vi "Bertta_v09_0.vi"() -> ()   [LabVIEW 2015]
panel:
  out "Started:":string
  in  "SHUTDOWN":bool
  in  "MASTER CONTROL":bool
  in  "Tab Control":T1(tab)
  in  "Read Seq":bool
  in  "Save Seq":bool
  in  "Configuration file":path=path "C:/Users/shresplab/Desktop/BerttaConfiguration.lvm" caption="Filename"
  in  "OK Button 2":bool
  out "Boolean":bool
  in  "User (initials)":string
  in  "Project name":string
  in  "Description":string
  out "Output file":string
  out "Sensor OK 6":bool
  out "Sensor OK 5":bool
  out "Sensor OK 4":bool
  out "Sensor OK 3":bool
  in  "OK Button":bool
  in  "Add comment":string
  out "PUMP 1":bool
  out "Target amount":dbl
  out "Scale weight":dbl
  out "Amount now":dbl
  out "Flow rate":dbl
  out "Time to target":dbl format="%<%H:%M:%S>t"
  out "Current step":dbl
  out "Target amount":dbl
  out "Amount now":dbl
  out "Tr":dbl
  out "Tj in":dbl
  out "Tj out":dbl
  out "T set":dbl
  out "Current step":i32
  out "RPM":dbl
  out "Torque 2":dbl
  out "Waveform Chart 5":dynamicdata(graph)
  out "Waveform Chart 6":dynamicdata(graph)
  out "Waveform Chart 7":dynamicdata(graph)
  out "Amount now":dbl
  out "Target amount":dbl
  out "Current step":dbl
  out "Time to target":dbl format="%<%H:%M:%S>t"
  out "Flow rate":dbl
  out "Amount now":dbl
  out "Scale weight":dbl
  out "Target amount":dbl
  out "PUMP 2":bool
  in  "Tab Control 2":T2(tab)
  out "Waveform Chart 3":dynamicdata(graph)
  out "Waveform Chart 8":dynamicdata(graph)
  out "Waveform Chart 11":dynamicdata(graph)
  out "Waveform Chart 9":dynamicdata(graph)
  out "Table":string[][](table)=[["14.8.2017 18.06.59", "0,000000", "417,670000", "-0,150000", "1,000000", "22,220000", "23,366837", "23,574959", "23,985852", "23,690000", "240,000000", "4,000000", "0,000000", "397,000000", "-397,000000", "1,000000"], ["14.8.2017 18.07.06", "0,000000", "417,640000", "-0,120000", "1,000000", "22,220000", "23,763115", "23,906257", "23,985694", "23,680000", "240,000000", "4,000000", "0,000000", "397,000000", "-397,000000", "1,000000"], ["14.8.2017 18.07.13", "0,000000", "417,640000", "-0,120000", "1,000000", "22,220000", "23,965922", "24,013440", "23,984906", "23,670000", "240,000000", "4,100000", "3,000000", "397,000000", "-397,000000", "1,000000"], ["14.8.2017 18.07.21", "0,000000", "417,640000", "-0,120000", "1,000000", "22,220000", "23,943860", "23,900110", "23,987113", "23,670000", "240,000000", "4,000000", "0,000000", "397,000000", "-397,000000", "1,000000"], ["14.8.2017 18.07.28", "0,000000", "417,640000", "-0,120000", "1,000000", "22,220000", "23,736328", "23,600018", "23,989004", "23,660000", "240,000000", "4,000000", "0,000000", "397,000000", "-397,000000", "1,000000"], ["14.8.2017 18.07.36", "0,000000", "417,640000", "-0,120000", "1,000000", "22,220000", "23,480910", "23,324538", "23,991053", "23,660000", "240,000000", "4,000000", "0,000000", "397,000000", "-397,000000", "1,000000"], ["14.8.2017 18.07.43", "0,000000", "417,640000", "-0,120000", "2,000000", "22,220000", "23,195579", "23,008270", "23,999093", "23,650000", "240,000000", "4,000000", "0,000000", "397,000000", "-397,000000", "1,000000"], ["14.8.2017 18.07.51", "0,000000", "417,650000", "-417,650000", "1,000000", "22,220000", "22,862541", "22,649021", "24,003979", "23,650000", "240,000000", "4,000000", "0,000000", "397,000000", "-397,000000", "2,000000"], ["14.8.2017 18.07.58", "0,000000", "417,640000", "0,010000", "1,000000", "22,220000", "22,541353", "22,354878", "24,005398", "23,650000", "240,000000", "4,000000", "0,000000", "397,000000", "-397,000000", "1,000000"], ["14.8.2017 18.08.06", "0,000000", "417,640000", "0,010000", "1,000000", "22,220000", "22,347931", "22,253738", "24,007605", "23,640000", "240,000000", "4,100000", "0,000000", "397,000000", "-397,000000", "1,000000"], ["14.8.2017 18.08.13", "0,000000", "417,640000", "0,010000", "1,000000", "22,220000", "22,329030", "22,302102", "24,006028", "23,640000", "240,000000", "4,000000", "0,000000", "395,820000", "-395,820000", "1,000000"], ["14.8.2017 18.08.20", "0,000000", "417,640000", "0,010000", "1,000000", "22,220000", "22,466849", "22,511320", "24,002403", "23,630000", "240,000000", "4,000000", "0,000000", "395,830000", "-0,010000", "1,000000"], ["14.8.2017 18.08.28", "0,000000", "417,640000", "0,010000", "1,000000", "22,220000", "22,707062", "22,835101", "24,000984", "23,620000", "240,000000", "4,000000", "0,000000", "395,830000", "-0,010000", "1,000000"], ["14.8.2017 18.08.35", "0,000000", "417,640000", "0,010000", "1,000000", "22,220000", "23,054104", "23,232979", "24,001299", "23,600000", "240,000000", "4,000000", "0,000000", "395,830000", "-0,010000", "1,000000"], ["14.8.2017 18.08.43", "0,000000", "417,640000", "0,010000", "1,000000", "22,220000", "23,412371", "23,522793", "24,002560", "23,590000", "240,000000", "4,000000", "0,000000", "395,820000", "0,000000", "1,000000"], ["14.8.2017 18.08.51", "0,000000", "417,640000", "0,010000", "1,000000", "22,220000", "23,596247", "23,656125", "24,003821", "23,580000", "240,000000", "4,000000", "0,000000", "395,820000", "0,000000", "1,000000"]]
  in  "T ext / T ext 2":enum32{"External 1", "External 2"}(radio)
  out "Sensor OK":bool
  in  "T fail":dbl=20.0
  out "Boolean 12":bool
  out "Boolean 7":bool
  out "Boolean 6":bool
  out "Boolean 5":bool
  out "Boolean 4":bool
  in  "?":bool
  in  "T manual setpoint":dbl=20.0
  in  "Lauda port":dbl=9.0
  in  "Manual select":enum32{"Tr", "Tj"}(radio)
  in  "TempSeq":dbl[][](array[numeric])=[[20.0, 40.0, 1.0, 30.0], [40.0, 50.0, 1.0, 30.0], [50.0, 20.0, 1.0, 30.0], [20.0, 20.0, 0.0, 20.0], [20.0, 20.0, 0.0, 20.0], [20.0, 20.0, 1000.0, 20.0]]
  out "T control":dbl
  out "Tr":dbl
  out "Tj in":dbl
  out "Tj out":dbl
  out "DT":dbl
  out "Elapsed":i32 format="%<%H:%M:%S>T"
  in  "PAUSE":bool
  out "Boolean 19":bool
  in  "Reset":bool
  in  "Treshold (Tset)":dbl=1.0
  in  "Tmax":dbl=199.0
  in  "Tmin":dbl=20.0
  out "Waveform Chart":dynamicdata(graph)
  out "T external 2":dbl
  in  "Xe":dbl=1.0
  in  "Ring":u16(ring) items=["SCALE 1", "SCALE 2", "SCALE 3"]
  out "Data out":dbl
  out "Port":i32=10
  in  "Radio Buttons":enum32{"Reglo Digital", "Reglo Analog", "PAM"}(radio)=enum."Reglo Analog"
  out "Speed":dbl
  out "mA":dbl format="%#_2g"
  in  "Port":i32=16
  out "RPM":dbl format="%#_2g"
  out "Boolean 18":bool
  out "Boolean 17":bool
  out "Boolean 16":bool
  out "Boolean 15":bool
  out "Boolean 14":bool
  out "Boolean 13":bool
  out "Boolean 11":bool
  out "Boolean 10":bool
  out "Boolean 9":bool
  out "Boolean 8":bool
  in  "PumpSeq":dbl[][](array[numeric])=[[3.0, 3.0, 7.0], [2.0, 2.0, 2.0], [4.0, 2.0, 100.0], [0.0, 0.0, 0.0], [0.0, 0.0, 0.0], [0.0, 0.0, 0.0], [0.0, 0.0, 0.0], [0.0, 0.0, 0.0], [0.0, 0.0, 0.0], [0.0, 0.0, 0.0], [0.0, 1.0, 0.0]]
  in  "?":bool
  out "Flow rate (g/min)":dbl
  out "Time (min)":dbl
  out "Target (g)":dbl
  out "Scale reading":dbl
  out "Step amount now":dbl
  out "Time to target":dbl format="%<%H:%M:%S>t"
  in  "Grams / min":dbl
  out "Waveform Chart 2":dynamicdata(graph)
  in  "?":bool
  out "Total amount now":dbl
  out "Total time":dbl
  out "Total amount target":dbl
  out "Boolean 20":bool
  in  "Reset 2":bool
  out "Waveform Chart 10":dynamicdata(graph)
  in  "Reset 3":bool
  out "Boolean 31":bool
  out "Total amount target 2":dbl
  out "Total time 2":dbl
  out "Boolean 30":bool
  out "Boolean 29":bool
  out "Boolean 28":bool
  out "Boolean 27":bool
  out "Boolean 26":bool
  out "Boolean 25":bool
  out "Boolean 24":bool
  out "Boolean 23":bool
  out "Boolean 22":bool
  out "Boolean 21":bool
  in  "PumpSeq 2":dbl[][](array[numeric])=[[3.0, 3.0, 7.0], [2.0, 2.0, 2.0], [4.0, 2.0, 100.0], [0.0, 0.0, 0.0], [0.0, 0.0, 0.0], [0.0, 0.0, 0.0], [0.0, 0.0, 0.0], [0.0, 0.0, 0.0], [0.0, 0.0, 0.0], [0.0, 0.0, 0.0], [0.0, 1.0, 0.0]]
  in  "Ring 2":u16(ring)=1 items=["SCALE 1", "SCALE 2", "SCALE 3"]
  out "Data out 2":dbl
  out "Port 3":i32=10
  in  "Radio Buttons 2":enum32{"Reglo Digital", "Reglo Analog", "PAM"}(radio)
  out "RPM":dbl format="%#_2g"
  in  "Port":i32=15
  out "mA":dbl format="%#_2g"
  out "Speed":dbl
  in  "?":bool
  in  "Grams / min":dbl
  out "Time (min)":dbl
  out "Target (g)":dbl
  out "Total amount now":dbl
  out "Time to target":dbl format="%<%H:%M:%S>t"
  in  "?":bool
  out "Step amount now":dbl
  out "Scale reading":dbl
  out "Flow rate (g/min)":dbl
  in  "Bypass select 2":enum32{"Remote", "Manual"}(radio)
  in  "Port":dbl=13.0
  out "RPM":dbl
  out "Torque":dbl
  in  "Set RPM":dbl(slide) scale=0.0..500.0
  out "Waveform Chart 4":dynamicdata(graph)
  out "DAQ 9217 (PT100)":errorcluster
  # "PUMP & SCALE 1"
  # "PUMP & SCALE 2"
  # "STEP"
  # "STEP"
  # "TOTAL"
  # "TOTAL"
  # "Temperature sensor:"
  # "Manual control:"
  # "Tinit     >    Tset       Min. time      Tfail"
  # "Manual control / end of sequence"
  # "Manual control"
  # "Secondary temperature sensor"
  # "Device communication"
  # "Grams    /   min"
  # "End of sequence"
  # "Manual control"
  # "Device communication"
  # "Pump configuration"
  # "Scale configuration"
  # "Grams    /   min"
  # "End of sequence"
  # "Manual control"
  # "Device communication"
  # "Pump configuration"
  # "Scale configuration"
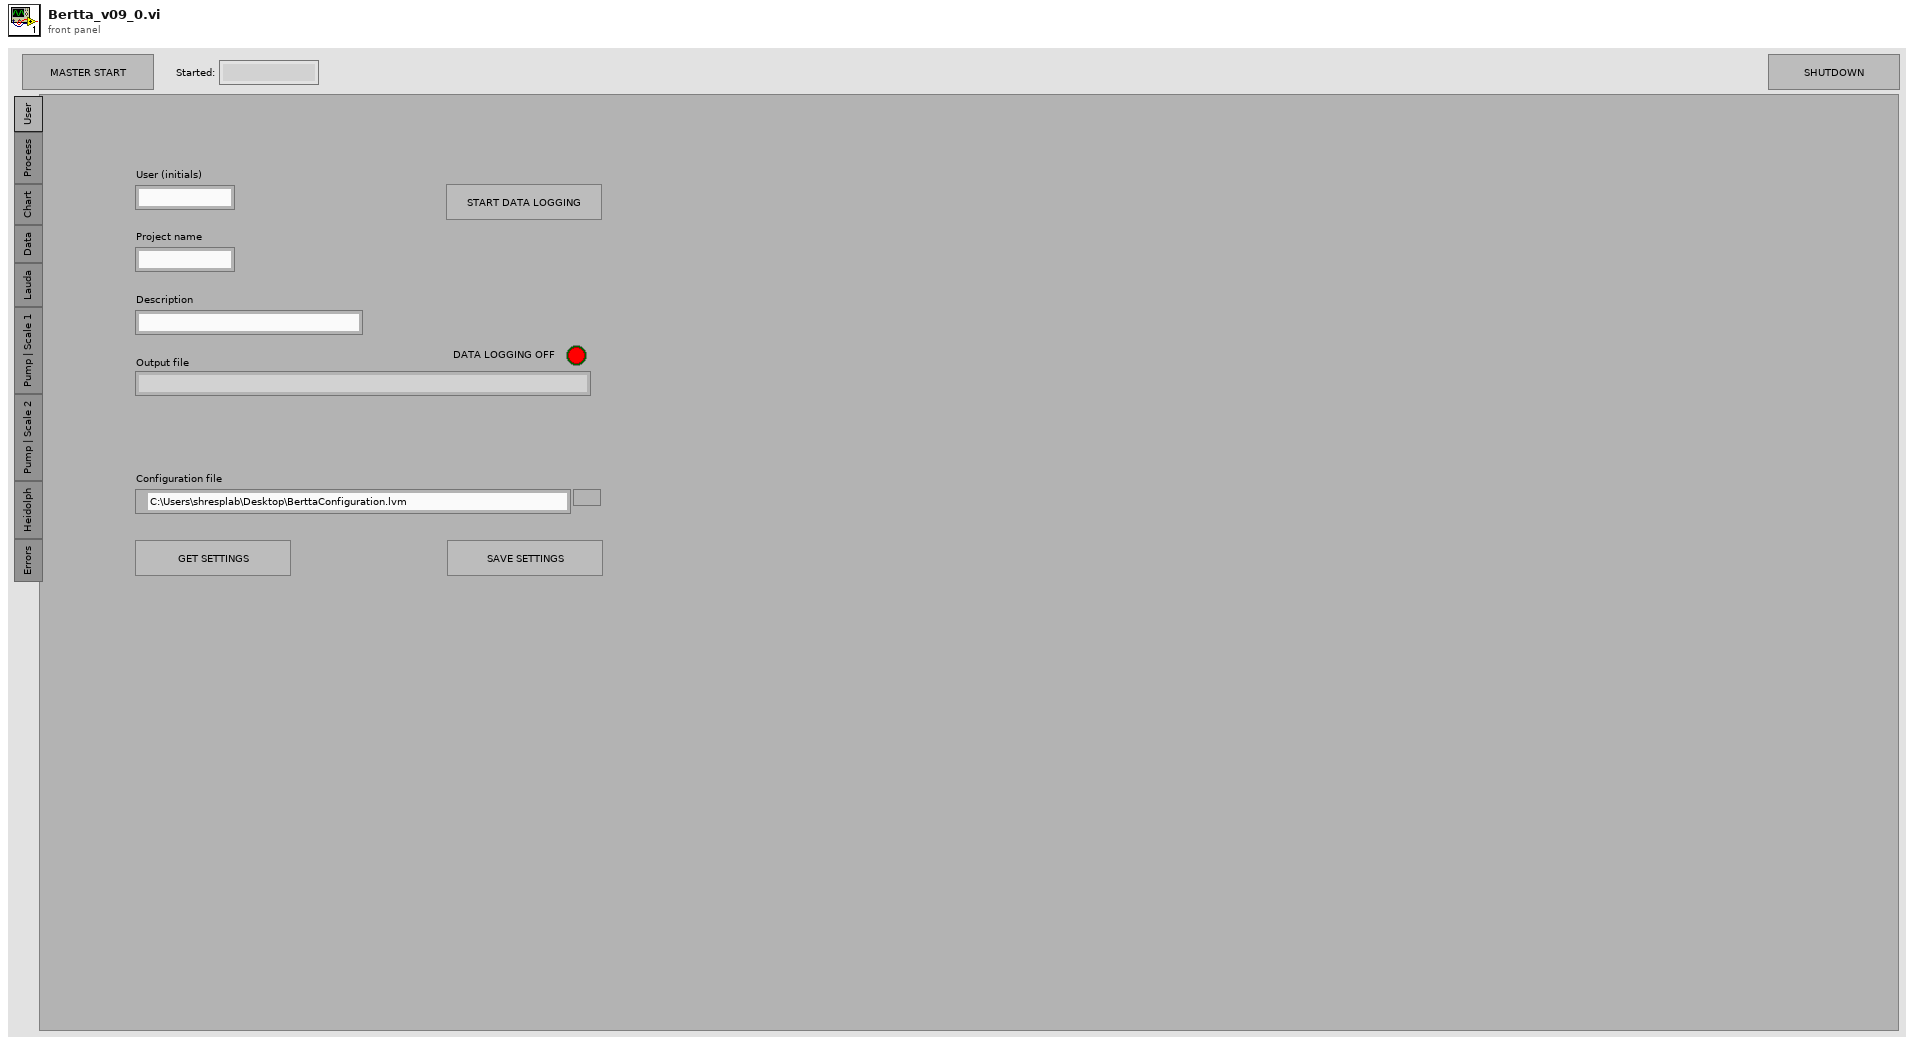
[diagram p1: front panel]
types:
  T1 = enum32{"User", "Process", "Chart", "Data", "Lauda", "Pump | Scale 1", "Pump | Scale 2", "Heidolph", "Errors"}
  T2 = enum32{"Temperatures", "Scale / Pump 1", "Scale / Pump 2", "RPM / torque"}
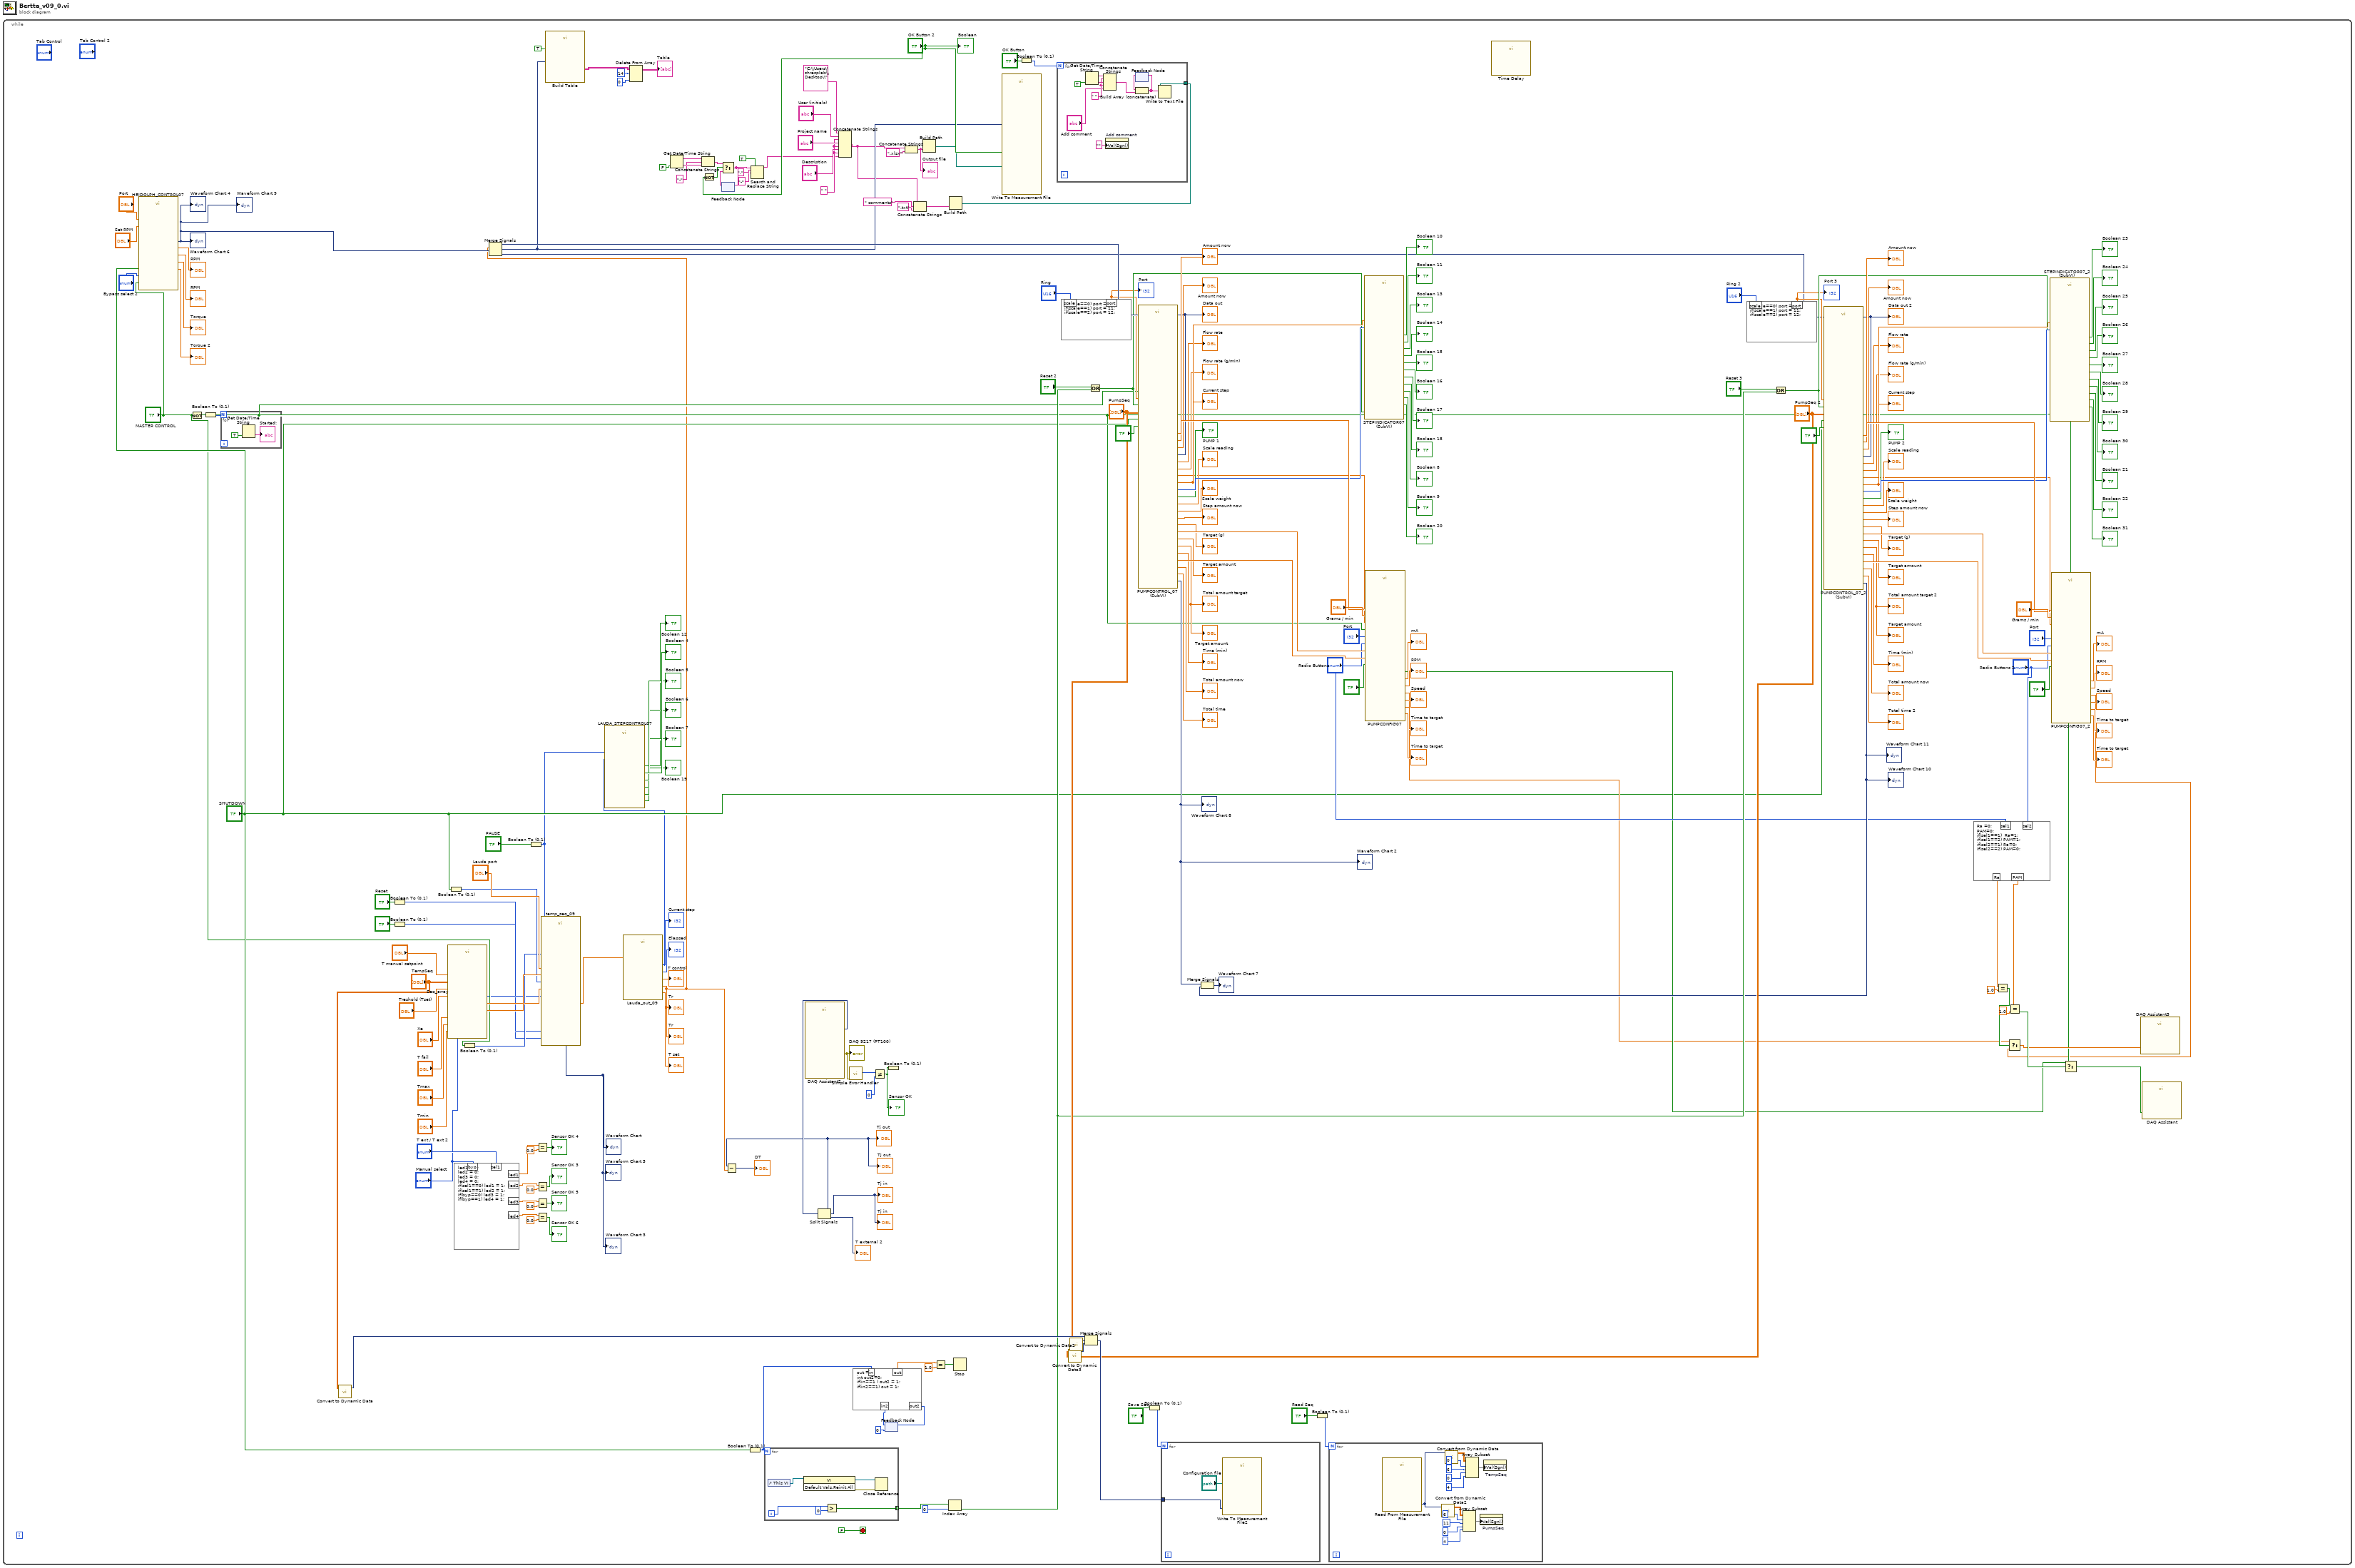
[diagram p0: block diagram]
diagram:
  n1 = while {
    stop <- FALSE stop-if-true
    w174 = " "
    n2 = call "HEIDOLPH_CONTROL07.vi"("master"="MASTER CONTROL", "shutdown"="SHUTDOWN", "Bypass select"="Bypass select 2", "Set RPM"="Set RPM", "Device port"="Port") -> ("Dynamic Data"=w185:dynamicdata, "RPM"=→"RPM":dbl, "RPM 2"=→"RPM":dbl, "Torque"=→"Torque":dbl, "Torque 2"=→"Torque 2":dbl)  [unwired: 2 in]
    "Waveform Chart 4" <- w185
    "Waveform Chart 6" <- w185
    "Waveform Chart 9" <- w185
    n3 = Not(x="MASTER CONTROL") -> (.not. x?=w165:bool)
    n4 = Boolean To (0,1)(Boolean=w165) -> (0, 1=w166:i16)
    n5 = for {
      N: w166 -> [_]
      n6 = Get Date/Time String(want seconds? (F)=TRUE) -> (time string=→"Started:":string)  [unwired: 2 in, 1 out]
    }
    n7 = call "Convert to Dynamic Data"("2D Array"="TempSeq") -> ("Dynamic Data Type"=w160:dynamicdata)  [unwired: 3 in]
    n8 = Boolean To (0,1)(Boolean="Reset") -> (0, 1=w13:i16)
    n9 = Boolean To (0,1)(Boolean="?") -> (0, 1=w15:i16)
    n10 = call "Seq_array.vi"("Tfail_manual"="T fail", "TempSeq in"="TempSeq", "Tmin"="Tmin", "Tmax"="Tmax", "Treshold (Tset)"="Treshold (Tset)", "T manual setpoint"="T manual setpoint", "Xe"="Xe") -> ("TimeParams"=w29:dbl[], "TempParams"=w30:dbl[])  [unwired: 3 in]
    n11 = Boolean To (0,1)(Boolean="SHUTDOWN") -> (0, 1=w25:i16)
    n12 = formula code="led1 = 0;\nled2 = 0;\nled3 = 0;\nled4 = 0;\nif(sel1==0) led1 = 1;\nif(sel1==1) led2 = 1;\nif(byp==0) led3 = 1;\nif(byp==1) led4 = 1;"("sel1"="T ext / T ext 2", "byp"="Manual select") -> ("led1"=w109:dbl, "led2"=w107:dbl, "led3"=w102:dbl, "led4"=w101:dbl)
    n13 = Boolean To (0,1)(Boolean="MASTER CONTROL") -> (0, 1=w23:i16)
    n14 = Boolean To (0,1)(Boolean="PAUSE") -> (0, 1=w19:i16)
    n15 = Equal?(x=w109, y=0.0) -> (x = y?=→"Sensor OK 4":bool)
    n16 = Equal?(x=w107, y=0.0) -> (x = y?=→"Sensor OK 3":bool)
    n17 = Equal?(x=w102, y=0.0) -> (x = y?=→"Sensor OK 5":bool)
    n18 = Equal?(x=w101, y=0.0) -> (x = y?=→"Sensor OK 6":bool)
    n19 = call "temp_seq_09.vi"("master"=w23, "shutdown"=w25, "Tr_orTj"="Manual select", "pause"=w19, "TempParams"=w30, "TimeParams"=w29, "port"="Lauda port", "reset"=w13, "manual"=w15) -> ("params"=w21:dbl[], "Waveform Chart"=→"Waveform Chart 3" →"Waveform Chart" →"Waveform Chart 5":dynamicdata)  [unwired: 3 in, 2 out]
    n20 = call "Lauda_out_09.vi"("params"=w21) -> ("Elapsed"=→"Elapsed":i32, "Tr"=w3:dbl, "Current step"=w2:i32, "T control"=→"T control":dbl, "T set"=→"T set":dbl)  [unwired: 6 in]
    "Tr" <- w3
    "Tr" <- w3
    "Current step" <- w2
    n21 = call "LAUDA_STEPCONTROL07.vi"("step"=w2, "pause"=w19) -> ("Boolean 13"=→"Boolean 19":bool, "Boolean 6"=→"Boolean 6":bool, "Boolean 5"=→"Boolean 5":bool, "Boolean 4"=→"Boolean 4":bool, "Boolean 7"=→"Boolean 7":bool, "Boolean 12"=→"Boolean 12":bool)  [unwired: 4 in]
    n22 = Get Date/Time String(want seconds? (F)=FALSE) -> (date string=w145:string, time string=w140:string)  [unwired: 2 in]
    n23 = Concatenate Strings(w145, "-" ("string"), w140) -> (w144:string)
    n24 = Not(x="OK Button 2") -> (.not. x?=w141:bool)
    n25 = feedback #1() -> (w143:string)  [unwired: 1 in]
    n26 = Select(t=w144, s=w141, f=w143) -> (s? t:f=w136:string)
    n27 = feedback-in #1(w136) -> ()
    n28 = Boolean To (0,1)(Boolean="SHUTDOWN") -> (0, 1=w115:i16)
    n29 = Search and Replace String(replace all?=TRUE ("replace all? (F)"), input string=w136, search string=".", replace string="-" ("replace string (\"\")")) -> (result string=w135:string)  [unwired: 4 in, 3 out]
    n30 = for {
      N: w115 -> [_]
      tunnel: [w254] -> w162 mode=indexing
      i -> [w256]
      n31 = control-ref of="This VI"() -> (w259:refnum<vi>)
      n32 = invoke class="VI" method="Default Vals.Reinit All"(reference=w259) -> (reference out=w257:refnum<vi>, error out=w258:errorcluster)  [unwired: 2 in, 1 out]
      n33 = Greater?(x=w256, y=0) -> (0:w254:bool)
      n34 = Close Reference(reference=w257, error in (no error)=w258) -> ()  [unwired: 1 out]
    }
    n35 = call "DAQ Assistant2"() -> ("data"=w8:dynamicdata, "error out"=w180:errorcluster)  [unwired: 17 in, 1 out]
    "DAQ 9217 (PT100)" <- w180
    n36 = Split Signals(w8) -> (w5:dynamicdata, →"Tj in" →"Tj in":dynamicdata, →"T external 2":dynamicdata)  [unwired: 3 in]
    "Tj out" <- w5
    "Tj out" <- w5
    n37 = Subtract(x=w5, y=w3) -> (x-y=→"DT":dynamicdata)
    n38 = Concatenate Strings("C:\\Users\\shresplab\\Desktop\\", "User (initials)", w174, "Project name", w174, "Description", w174, w135) -> (w125:string)
    n39 = call <vilib>:"Simple Error Handler.vi"("error in (no error)"=w180) -> ("code out"=w179:i32)  [unwired: 4 in, 4 out]
    n40 = Not Equal?(x=w179, y=0) -> (x != y?=w152:bool)
    "Sensor OK" <- w152
    n41 = feedback #2(0) -> (w113:i32)
    n42 = formula code="out = 0;\nint out2=0;\nif(in==1 ) out2 = 1;\nif(in2==1) out = 1;"("in"=w115, "in2"=w113) -> ("out"=w117:dbl, "out2"=w114:i32)
    n43 = feedback-in #2(w114) -> ()
    n44 = Boolean To (0,1)(Boolean=w152) -> ()  [unwired: 1 out]
    n45 = Concatenate Strings(w125, ".xlsx") -> (w128:string)
    "Output file" <- w128
    n46 = Concatenate Strings(w125, " comments" ("string"), ".txt" ("string")) -> (w122:string)
    n47 = Build Path(name or relative path=w128) -> (appended path=w126:path)  [unwired: 1 in]
    n48 = Equal?(x=w117, y=1.0) -> (x = y?=w116:bool)
    n49 = Index Array(array=w162, index=0) -> (element=w54:bool)
    n50 = Build Path(name or relative path=w122) -> (appended path=w121:path)  [unwired: 1 in]
    n51 = Stop(stop? (T)=w116) -> ()
    n52 = Boolean To (0,1)(Boolean="OK Button") -> (0, 1=w120:i16)
    n53 = for {
      N: w120 -> [_]
      tunnel: w121 -> [w231]
      w235 = " " ("string")
      n54 = Get Date/Time String(want seconds? (F)=TRUE) -> (date string=w238:string, time string=w236:string)  [unwired: 2 in]
      n55 = Concatenate Strings(w238, w235, w236, w235, "Add comment") -> (w234:string)
      n56 = property on="Add comment" class="Str"("Val(Sgnl)"="" ("Value (Signaling)")) -> ()  [unwired: 2 in, 2 out]
      n57 = feedback #3() -> (w233:string[])  [unwired: 1 in]
      n58 = Build Array (concatenate)(w233, w234) -> (w232:string[])
      n59 = feedback-in #3(w232) -> ()
      n60 = Write to Text File(file (use dialog)=w231, text=w232) -> ()  [unwired: 2 in, 3 out]
    }
    n61 = formula code="if(scale==0) port = 10;\nif(scale==1) port = 11;\nif(scale==2) port = 12;"("scale"="Ring") -> ("port"=w147:dbl)
    "Port" <- w147
    n62 = call "Convert to Dynamic Data3"("2D Array"="PumpSeq 2") -> ("Dynamic Data Type"=w53:dynamicdata)  [unwired: 3 in]
    n63 = call "Convert to Dynamic Data2"("2D Array"="PumpSeq") -> ("Dynamic Data Type"=w159:dynamicdata)  [unwired: 3 in]
    n64 = Merge Signals(w160, w159, w53) -> (w158:dynamicdata)
    n65 = Or(x="Reset 2", y=w54) -> (x .or. y?=w151:bool)
    n66 = call "PUMPCONTROL_07 (SubVI).vi"("Port"=w147, "Pause"="MASTER CONTROL", "Master start"="?", "shutdown"="SHUTDOWN", "Seq in"="PumpSeq", "reset"=w151) -> ("Amount now"=→"Amount now":dbl, "Amount now 2"=→"Amount now":dbl, "Flow rate out"=w170:dbl, "Step amount now"=→"Step amount now":dbl, "Total amount now"=→"Total amount now":dbl, "Total time"=→"Total time":dbl, "Numeric 2"=w223:i16, "PUMP 1"=→"PUMP 1":bool, "Numeric"=w220:dbl, "Flow rate"=→"Flow rate":dbl, "Dynamic Data"=w186:dynamicdata, "Target amount"=→"Target amount":dbl, "Time (min) 2"=w224:dbl, "Target amount 2"=→"Total amount target" →"Target amount":dbl, "Scale reading"=→"Scale reading":dbl, "Flow rate (g/min)"=→"Flow rate (g/min)":dbl, "Target (g) 2"=w225:dbl, "Target (g)"=→"Target (g)":dbl, "Time (min)"=→"Time (min)":dbl, "Waveform Chart 2"=w36:dynamicdata, "Scale weight"=→"Scale weight":dbl, "Amount (g)"=w226:dbl)
    "Waveform Chart 2" <- w36
    "Current step" <- w220
    "Data out" <- w186
    "Waveform Chart 8" <- w36
    n67 = Boolean To (0,1)(Boolean="Save Seq") -> (0, 1=w157:i16)
    n68 = for {
      N: w157 -> [_]
      tunnel: w158 -> [w253]
      n69 = call "Write To Measurement File2"("Signals"=w253, "Filename"="Configuration file") -> ()  [unwired: 15 in, 3 out]
    }
    n70 = Boolean To (0,1)(Boolean="Read Seq") -> (0, 1=w154:i16)
    n71 = for {
      N: w154 -> [_]
      n72 = call "Read From Measurement File"() -> ("Signals"=w241:dynamicdata)  [unwired: 6 in, 5 out]
      n73 = call "Convert from Dynamic Data2"("Dynamic Data Type"=w241) -> ("Array"=w240:dbl[][])  [unwired: 3 in]
      n74 = call "Convert from Dynamic Data"("Dynamic Data Type"=w241) -> ("Array"=w249:dbl[][])  [unwired: 3 in]
      n75 = Array Subset(array=w240, index (row)=6 ("index"), length (row)=11 ("length"), index (col)=0 ("index"), length (col)=4 ("length")) -> (w239:dbl[][])
      n76 = Array Subset(array=w249, index (row)=0 ("index"), length (row)=6 ("length"), index (col)=0 ("index"), length (col)=4 ("length")) -> (w246:dbl[][])
      n77 = property on="PumpSeq" class="Arr (strict)"("Val(Sgnl)"=w239) -> ()  [unwired: 2 in, 2 out]
      n78 = property on="TempSeq" class="Arr (strict)"("Val(Sgnl)"=w246) -> ()  [unwired: 2 in, 2 out]
    }
    n79 = call "STEPINDICATOR07 (SubVI).vi"("Numeric"=w220, "Numeric 2"=w223, "Reset"=w151) -> ("Boolean 18"=→"Boolean 18":bool, "Boolean 8"=→"Boolean 8":bool, "Boolean 9"=→"Boolean 9":bool, "Boolean 17"=→"Boolean 17":bool, "Boolean 10"=→"Boolean 10":bool, "Boolean 16"=→"Boolean 16":bool, "Boolean 11"=→"Boolean 11":bool, "Boolean 15"=→"Boolean 15":bool, "Boolean 14"=→"Boolean 14":bool, "Boolean 13"=→"Boolean 13":bool, "Boolean 19"=→"Boolean 20":bool)  [unwired: 2 in]
    n80 = call "PUMPCONFIG07.vi"(0:"?", "Radio Buttons"="Radio Buttons", "Bypass (g/min)"="Grams / min", "Target (g) in"=w225, "Amount (g)"=w226, "Time (min) in"=w224, "Flow rate in"=w170, "OK Button"="MASTER CONTROL", "Port"="Port") -> ("Time to target 2"=→"Time to target":dbl, "Time to target"=→"Time to target":dbl, "mA"=→"mA":dbl, "signal"=w40:dbl, "Speed"=→"Speed":dbl, "RPM"=→"RPM":dbl, "Array"=w42:bool[])
    n81 = call "Time Delay"() -> ()  [unwired: 11 in, 1 out]
    n82 = formula code="if(scale==0) port = 10;\nif(scale==1) port = 11;\nif(scale==2) port = 12;"("scale"="Ring 2") -> ("port"=w55:dbl)
    "Port 3" <- w55
    n83 = Or(x="Reset 3", y=w54) -> (x .or. y?=w58:bool)
    n84 = call "PUMPCONTROL_07_2 (SubVI).vi"("Port"=w55, "Pause"="MASTER CONTROL", "Master start"="?", "shutdown"="SHUTDOWN", "Seq in"="PumpSeq 2", "reset"=w58) -> ("Amount now"=→"Amount now":dbl, "Amount now 2"=→"Amount now":dbl, "Flow rate out"=w62:dbl, "Step amount now"=→"Step amount now":dbl, "Total amount now"=→"Total amount now":dbl, "Total time"=→"Total time 2":dbl, "Numeric 2"=w94:i16, "PUMP 1"=→"PUMP 2":bool, "Numeric"=w91:dbl, "Flow rate"=→"Flow rate":dbl, "Dynamic Data"=w34:dynamicdata, "Target amount"=→"Target amount":dbl, "Time (min) 2"=w95:dbl, "Target amount 2"=→"Total amount target 2" →"Target amount":dbl, "Scale reading"=→"Scale reading":dbl, "Flow rate (g/min)"=→"Flow rate (g/min)":dbl, "Target (g) 2"=w96:dbl, "Target (g)"=→"Target (g)":dbl, "Time (min)"=→"Time (min)":dbl, "Waveform Chart 2"=w51:dynamicdata, "Scale weight"=→"Scale weight":dbl, "Amount (g)"=w97:dbl)
    "Waveform Chart 10" <- w51
    "Current step" <- w91
    "Data out 2" <- w34
    "Waveform Chart 11" <- w51
    n85 = Merge Signals(w186, w3, w185, w34) -> (w132:dynamicdata)
    n86 = call "Build Table"("Include time data"=TRUE, "Signals"=w132) -> ("Table"=w131:string[][])  [unwired: 3 in, 6 out]
    n87 = Delete From Array(array=w131, length=14, index (col)=0 ("index (row)")) -> (array with subset deleted=→"Table":string[][])  [unwired: 1 in, 1 out]
    n88 = call "Write To Measurement File"("Signals"=w132, "Enable"="OK Button 2", "Filename"=w126) -> ()  [unwired: 14 in, 3 out]
    n89 = Merge Signals(w36, w51) -> (→"Waveform Chart 7":dynamicdata)
    n90 = formula code="Ra =0;\nPAM=0;\nif(sel1==1)  Ra=1;\nif(sel1==2) PAM=1;\nif(sel2==1) Ra=0;\nif(sel2==2) PAM=0;"("sel1"="Radio Buttons", "sel2"="Radio Buttons 2") -> ("Ra"=w48:dbl, "PAM"=w45:dbl)
    n91 = Equal?(x=w48, y=1.0) -> (x = y?=w44:bool)
    n92 = Equal?(x=w45, y=1.0) -> (x = y?=w43:bool)
    n93 = call "STEPINDICATOR07_2 (SubVI).vi"("Numeric"=w91, "Numeric 2"=w94, "Reset"=w58) -> ("Boolean 18"=→"Boolean 30":bool, "Boolean 8"=→"Boolean 21":bool, "Boolean 9"=→"Boolean 22":bool, "Boolean 17"=→"Boolean 29":bool, "Boolean 10"=→"Boolean 23":bool, "Boolean 16"=→"Boolean 28":bool, "Boolean 11"=→"Boolean 24":bool, "Boolean 15"=→"Boolean 27":bool, "Boolean 14"=→"Boolean 26":bool, "Boolean 13"=→"Boolean 25":bool, "Boolean 19"=→"Boolean 31":bool)  [unwired: 2 in]
    n94 = call "PUMPCONFIG07_2.vi"(0:"?", "Radio Buttons"="Radio Buttons 2", "Bypass (g/min)"="Grams / min", "Target (g) in"=w96, "Amount (g)"=w97, "Time (min) in"=w95, "Flow rate in"=w62, "OK Button"="MASTER CONTROL", "Port"="Port") -> ("Time to target 2"=→"Time to target":dbl, "Time to target"=→"Time to target":dbl, "mA"=→"mA":dbl, "signal"=w37:dbl, "Speed"=→"Speed":dbl, "RPM"=→"RPM":dbl, "Array"=w38:bool[])
    n95 = Select(t=w40, s=w44, f=w37) -> (s? t:f=w39:dbl)
    n96 = Select(t=w42, s=w43, f=w38) -> (s? t:f=w41:bool[])
    n97 = call "DAQ Assistant3"("data"=w39) -> ()  [unwired: 17 in, 2 out]
    n98 = call "DAQ Assistant"("data"=w41) -> ()  [unwired: 17 in, 2 out]
    "Boolean" <- "OK Button 2"
  }
